vi "PDash Rename Module.vi"(8 "error in":errorcluster, 10 "Current Selection":T1, 11 "Project":refnum<class "Project.lvclass">) -> (0 "error out":errorcluster)   [LabVIEW 2020, in "Panther Dashboard.lvlib"]
doc: "Panther Dashboard DQMH Rename Module"
uses:
  Panther Dashboard.lvlib
  Controls/Cancel.ctl
  Controls/Continue.ctl
  Class/Project/Project.lvclass
  Class/Library/Library.lvclass
  C:/GitClones/PantherDashboard/src/LabVIEW/Panther Dashboard/Class/LabVIEWItem/LabVIEWItem.lvclass
  Class/VI/VI.lvclass
  Class/Library/Library.lvclass/Library.ctl
  Class/LabVIEWItem/LabVIEWItem.lvclass/LabVIEWItem.ctl
  <vilib>/Delacor/Delacor QMH/Libraries/_Scripting Support/Module Info--cluster.ctl
  <vilib>/Delacor/Delacor QMH/Libraries/_Scripting Support/Module Type--enum.ctl
  Class/Project/Project.lvclass/Project.ctl
  Class/Library/Read Library Ref.vi
  Class/LabVIEWItem/Read Item Name.vi
  Class/Project/Read Main App Inst Ref.vi
  Class/Project/Read Project Ref.vi
  <vilib>/Delacor/Delacor QMH/Libraries/_Scripting Support/dqmh_lib_DQMH Scripting Support.lvlib
panel:
  out "Selected Module":string caption="Current Selection:"
  in  "New Module":string caption="New Name"
  in  "Continue":T2
  in  "Cancel":T3
  # "Note: To Select the DQMH Default UIs, click the Gear Icon on the Panther Dashboard\nMain UI, and Uncheck the 'Use Panther Dashboard UIs' checkbox."
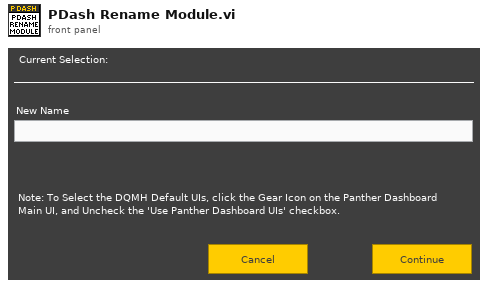
[diagram p1: front panel]
types:
  T1 = cluster{"Library":refnum<class "Library.lvclass">, "VI":refnum<class "VI.lvclass">}
  T2 = typedef "Continue.ctl" = bool
  T3 = typedef "Cancel.ctl" = bool
  T4 = typedef "dqmh_lib_DQMH Scripting Support.lvlib/Module Info--cluster.ctl" = cluster{"Name":string, "Library":refnum<vi>, "Library Owning App":refnum<vi>, "Library Owning Folder":path, "Module Type":T5, "Public API Requests Folder":refnum<vi>, "Public API Requests Arguments Folder":refnum<vi>, "Broadcasts Folder":refnum<vi>, "Broadcasts Arguments Folder":refnum<vi>, "Obtain Broadcast Events VI":refnum<vi>, "Destroy Broadcast Events VI":refnum<vi>, "Obtain Request Events VI":refnum<vi>, "Destroy Request Events VI":refnum<vi>, "Request Events Cluster CTL":refnum<vi>, "Broadcast Events Cluster CTL":refnum<vi>, "Module Timeout VI":refnum<vi>, "Module Name VI":refnum<vi>, "Status Updated VI":refnum<vi>, "Module Not Running Error Constant VI":refnum<vi>}
  T5 = typedef "dqmh_lib_DQMH Scripting Support.lvlib/Module Type--enum.ctl" = enum16{"Singleton", "Cloneable"}
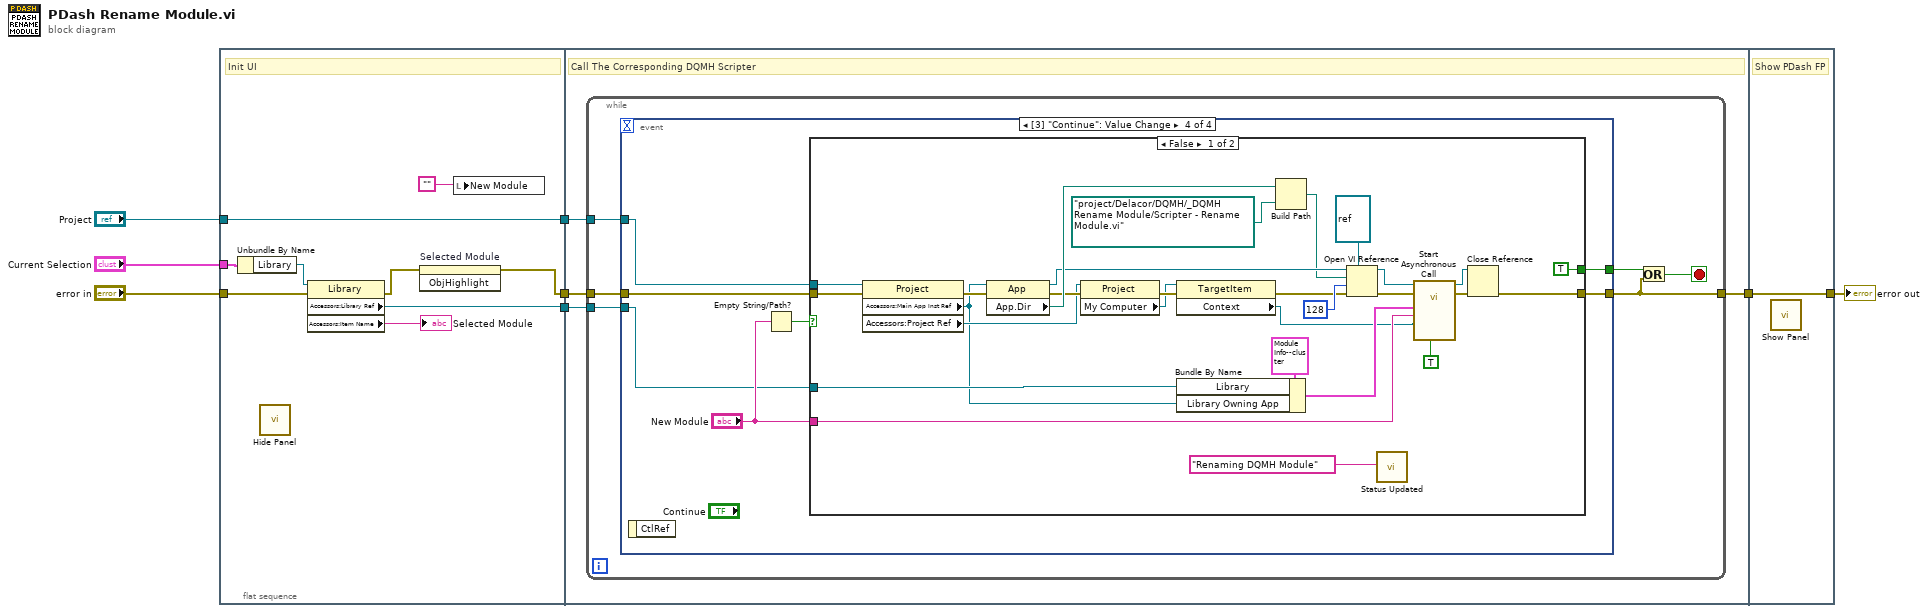
[diagram p0: block diagram]
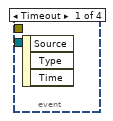
[diagram p2: hidden frame]
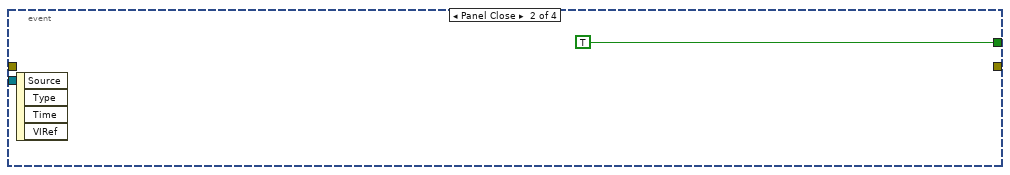
[diagram p3: hidden frame]
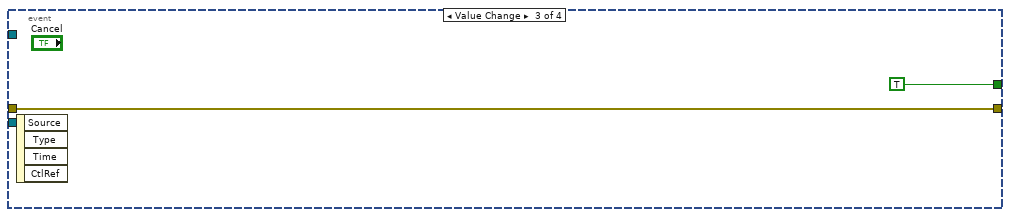
[diagram p4: hidden frame]
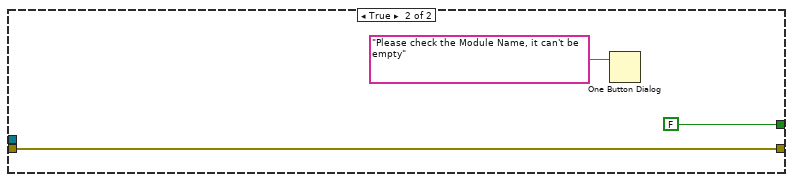
[diagram p5: hidden frame]
diagram:
  n1 = flat-sequence {
    tunnel: "Project" -> [w15]
    tunnel: [w15] -> w3
    tunnel: "error in" -> [w17]
    tunnel: [w9] -> w5
    tunnel: "Current Selection" -> [w14]
    tunnel: [w11] -> w1
    tunnel: [w21] -> w8
    tunnel: w3 -> [w19]
    tunnel: w5 -> [w20]
    tunnel: w1 -> [w18]
    tunnel: [w69] -> w7
    tunnel: w8 -> [w69]
    frame #0 {
      # "Init UI"
      n2 = Unbundle By Name(w14) -> ("Library"=w13:refnum<class "Library.lvclass">)
      n3 = call "Hide Panel.vi"() -> ()  [unwired: 11 in, 1 out]
      n4 = property class="Library"(reference=w13, error in=w17) -> (error out=w16:errorcluster, "Accessors:Library Ref"=w11:refnum<vi>, "Accessors:Item Name"=→"Selected Module":string)  [unwired: 1 out]
      n5 = invoke on="Selected Module" class="Str" method="ObjHighlight"(error in=w16) -> (error out=w9:errorcluster)  [unwired: 2 in, 2 out]
      n6 = local write "New Module"("") -> ()
    }
    frame #1 {
      # "Call The Corresponding DQMH Scripter"
      n7 = while {
        tunnel: [w22] -> w21
        tunnel: w19 -> [w25]
        tunnel: w20 -> [w27]
        tunnel: w18 -> [w24]
        stop <- w23 stop-if-true
        n8 = event shown="[3] \"Continue\": Value Change" {
          selector: _ -> [_ _ _ _]
          dyn-events: _ -> [_ _ _ _]
          timeout: _ -> [_ _ _ _]
          tunnel: [_ TRUE TRUE w31] -> w26
          tunnel: [_ _ w29 w33] -> w22
          tunnel: w25 -> [_ _ _ w36]
          tunnel: w27 -> [_ _ w29 w35]
          tunnel: w24 -> [_ _ _ w34]
          event Timeout {
            n9 = event-data() -> ()  [unwired: 1 in, 3 out]
          }
          event Panel Close {
            n10 = event-data() -> ()  [unwired: 1 in, 4 out]
          }
          event Value Change {
            n11 = event-data() -> ()  [unwired: 1 in, 4 out]
          }
          event Value Change {
            n12 = event-data() -> ()  [unwired: 1 in, 1 out]
            n13 = Empty String/Path?(string/path="New Module") -> (empty?=w32:bool)
            n14 = case shown="False" w32 {
              tunnel: "New Module" -> [w65 _]
              tunnel: w36 -> [w64 _]
              tunnel: w35 -> [w63 w67]
              tunnel: w34 -> [w62 _]
              tunnel: [w61 w67] -> w33
              tunnel: [TRUE FALSE] -> w31
              frame False {
                n15 = property class="Project"(reference=w64, error in=w63) -> (error out=w54:errorcluster, "Accessors:Main App Inst Ref"=w38:refnum<vi>, "Accessors:Project Ref"=w43:refnum<vi>)  [unwired: 1 out]
                n16 = property class="App"(reference=w38, error in=w54) -> (reference out=w58:refnum<vi>, error out=w53:errorcluster, "App.Dir"=w59:path)
                n17 = property class="Project"(reference=w43, error in=w53) -> (error out=w44:errorcluster, "My Computer"=w41:refnum<vi>)  [unwired: 1 out]
                n18 = property class="TargetItem"(reference=w41, error in=w44) -> (error out=w42:errorcluster, "Context"=w40:refnum<vi>)  [unwired: 1 out]
                n19 = Bundle By Name(cluster=T4 {"Name"="", "Library"=refnum, "Library Owning App"=refnum, "Library Owning Folder"=path "", "Module Type"=enum."Singleton", "Public API Requests Folder"=refnum, "Public API Requests Arguments Folder"=refnum, "Broadcasts Folder"=refnum, "Broadcasts Arguments Folder"=refnum, "Obtain Broadcast Events VI"=refnum, "Destroy Broadcast Events VI"=refnum, "Obtain Request Events VI"=refnum, "Destroy Request Events VI"=refnum, "Request Events Cluster CTL"=refnum, "Broadcast Events Cluster CTL"=refnum, "Module Timeout VI"=refnum, "Module Name VI"=refnum, "Status Updated VI"=refnum, "Module Not Running Error Constant VI"=refnum} ("Module Info in"), "Library"=w62, "Library Owning App"=w38) -> (w56:T4)
                n20 = Build Path(base path=w59, name or relative path=path "project/Delacor/DQMH/_DQMH Rename Module/Scripter - Rename Module.vi") -> (appended path=w55:path)
                n21 = Open VI Reference(type specifier VI Refnum (for type only)=refnum<vi> refnum, application reference (local)=w58, vi path=w55, options=128, error in (no error)=w42) -> (vi reference=w60:refnum<vi>, error out=w51:errorcluster)  [unwired: 1 in]
                n22 = call "Status Updated.vi"("Status"="Renaming DQMH Module") -> ()  [unwired: 10 in, 1 out]
                n23 = call-by-ref "Start Asynchronous Call"(reference=w60, error in=w51, "Show Progress? (F)"=TRUE, "My Computer"=w40, "New Module Name"=w65, "Module Info in"=w56) -> (reference out=w57:refnum<vi>, error out=w52:errorcluster)  [unwired: 6 in, 2 out]
                n24 = Close Reference(reference=w57, error in (no error)=w52) -> (error out=w61:errorcluster)
              }
              frame True {
                n25 = One Button Dialog(message="Please check the Module Name, it can't be empty") -> ()  [unwired: 1 in, 1 out]
              }
            }
          }
        }
        n26 = Or(x=w26, y=w22) -> (x .or. y?=w23:bool)
      }
    }
    frame #2 {
      # "Show PDash FP"
      n27 = call "Show Panel.vi"() -> ()  [unwired: 11 in, 1 out]
    }
  }
  "error out" <- w7
